vi "IMAQ_Attribute2Control_Dbl.vi"(3 "error in (no error)":errorcluster, 4 "IMAQ Attribute":variant, 5 "Refnum (Dbl)":refnum<vi>) -> (0 "error out":errorcluster, 1 "dup IMAQ Attribute":variant)   [LabVIEW 2012, in "HGF_VisionTools.lvlib"]
doc: "This Polymorphic VI set IMAQ control properties of type double according to variant inputp value and its attribute."
uses:
  HGF_VisionTools.lvlib
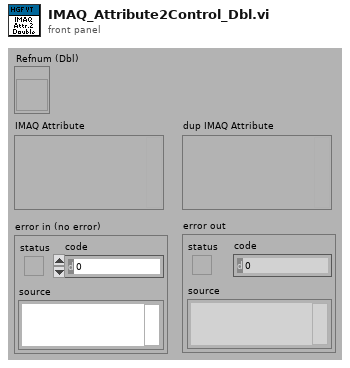
[diagram p1: front panel]
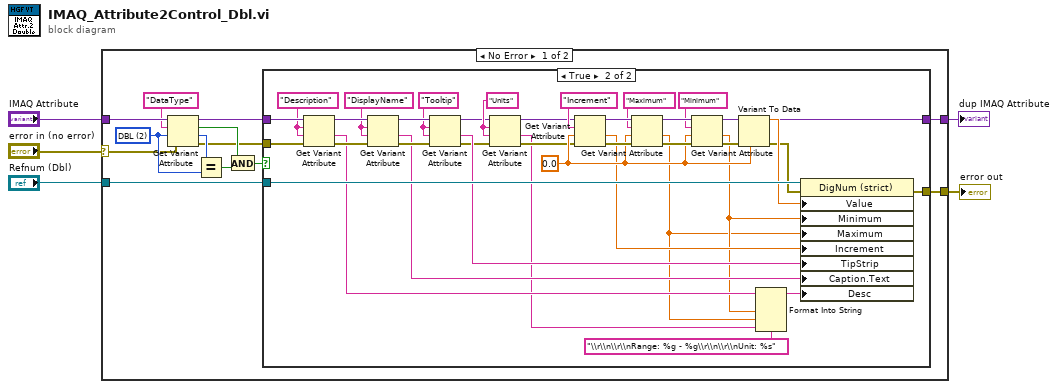
[diagram p0: block diagram]
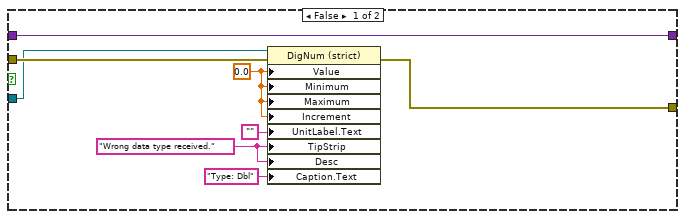
[diagram p2: hidden frame]
diagram:
  n1 = case shown="No Error" "error in (no error)" {
    selector: "error in (no error)" -> [w11 w65]
    tunnel: "IMAQ Attribute" -> [w18 w64]
    tunnel: "Refnum (Dbl)" -> [w6 _]
    tunnel: [w8 w65] -> w2
    tunnel: [w7 w64] -> w1
    frame No Error {
      w15 = u32 2 items=["U32", "I64", "DBL", "String", "Enum", "Bool", "Command"] ("Type")
      n2 = Get Variant Attribute(Variant=w18, name="DataType", default value (empty Variant)=w15, error in=w11) -> (duplicate Variant=w10:variant, found=w14:bool, value=w16:u32, error out=w9:errorcluster)
      n3 = Equal?(x=w16, y=w15) -> (x = y?=w13:bool)
      n4 = And(x=w14, y=w13) -> (x .and. y?=w12:bool)
      n5 = case shown="True" w12 {
        tunnel: w10 -> [w26 w63]
        tunnel: w9 -> [w25 w62]
        tunnel: w6 -> [w23 w61]
        tunnel: [w24 w41] -> w8
        tunnel: [w26 w40] -> w7
        frame False {
          w20 = "Wrong data type received." ("Tip Strip")
          w22 = 0.0 ("Value")
          n6 = property class="DigNum (strict)"(reference=w23, error in=w25, "Value"=w22, "Minimum"=w22, "Maximum"=w22, "Increment"=w22, "UnitLabel.Text"="", "TipStrip"=w20, "Desc"=w20, "Caption.Text"="Type: Dbl") -> (error out=w24:errorcluster)  [unwired: 1 out]
        }
        frame True {
          w39 = "Units" ("name")
          w46 = 0.0 ("Value")
          w43 = "Tooltip" ("name")
          w33 = "Description" ("name")
          w32 = "DisplayName" ("name")
          n7 = Get Variant Attribute(Variant=w63, name=w33, default value (empty Variant)=w33, error in=w62) -> (duplicate Variant=w54:variant, value=w42:string, error out=w55:errorcluster)  [unwired: 1 out]
          n8 = Get Variant Attribute(Variant=w54, name=w32, default value (empty Variant)=w32, error in=w55) -> (duplicate Variant=w53:variant, value=w34:string, error out=w56:errorcluster)  [unwired: 1 out]
          n9 = Get Variant Attribute(Variant=w53, name=w43, default value (empty Variant)=w43, error in=w56) -> (duplicate Variant=w37:variant, value=w44:string, error out=w38:errorcluster)  [unwired: 1 out]
          n10 = Get Variant Attribute(Variant=w37, name=w39, default value (empty Variant)=w39, error in=w38) -> (duplicate Variant=w36:variant, value=w28:string, error out=w35:errorcluster)  [unwired: 1 out]
          n11 = Get Variant Attribute(Variant=w36, name="Increment", default value (empty Variant)=w46, error in=w35) -> (duplicate Variant=w59:variant, value=w45:dbl, error out=w60:errorcluster)  [unwired: 1 out]
          n12 = Get Variant Attribute(Variant=w59, name="Maximum", default value (empty Variant)=w46, error in=w60) -> (duplicate Variant=w57:variant, value=w29:dbl, error out=w58:errorcluster)  [unwired: 1 out]
          n13 = Get Variant Attribute(Variant=w57, name="Minimum", default value (empty Variant)=w46, error in=w58) -> (duplicate Variant=w40:variant, value=w30:dbl, error out=w49:errorcluster)  [unwired: 1 out]
          n14 = Variant To Data(error in=w49, type=w46, Variant=w40) -> (data=w48:dbl, error out=w47:errorcluster)
          n15 = Format Into String(format string="\\r\\n\\r\\nRange: %g - %g\\r\\n\\r\\nUnit: %s", initial string=w42, w30, w29, w28) -> (resulting string=w31:string)  [unwired: 1 in, 1 out]
          n16 = property class="DigNum (strict)"(reference=w61, error in=w47, "Value"=w48, "Minimum"=w30, "Maximum"=w29, "Increment"=w45, "TipStrip"=w44, "Caption.Text"=w34, "Desc"=w31) -> (error out=w41:errorcluster)  [unwired: 1 out]
        }
      }
    }
    frame Error {
    }
  }
  "error out" <- w2
  "dup IMAQ Attribute" <- w1
